vi "Normalize Min To Max.vi"(2 "Max":dbl=1.0, 7 "Y":dbl[](array[numeric])) -> (8 "Ynorm":dbl[](array[numeric]))   [LabVIEW 2020]
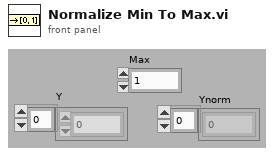
[diagram p1: front panel]
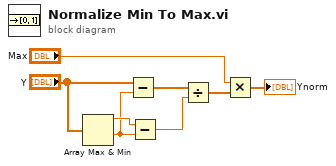
[diagram p0: block diagram]
diagram:
  n1 = Array Max & Min(array="Y") -> (max value=w5:dbl, min value=w4:dbl)  [unwired: 2 out]
  n2 = Subtract(x="Y", y=w4) -> (x-y=w6:dbl[])
  n3 = Subtract(x=w5, y=w4) -> (x-y=w3:dbl)
  n4 = Divide(x=w6, y=w3) -> (x/y=w8:dbl[])
  n5 = Multiply(x="Max", y=w8) -> (x*y=→"Ynorm":dbl[])
